vi "RadiusToBoundingBox.vi"(11 "Radius":i32) -> (3 "Array":i32[](array[numeric]))   [LabVIEW 2014]
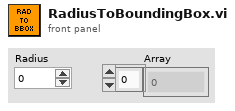
[diagram p1: front panel]
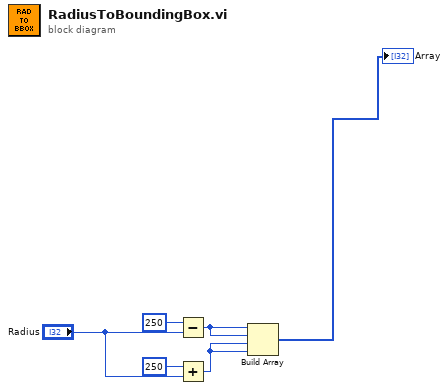
[diagram p0: block diagram]
diagram:
  n1 = Subtract(x=250, y="Radius") -> (x-y=w4:i32)
  n2 = Add(x=250, y="Radius") -> (x+y=w5:i32)
  n3 = Build Array(w4, w4, w5, w5) -> (→"Array":i32[])
